vi "T Test.vi"(6 "alternative hypothesis":i32(ring) items=["mean(pop) != mean"=0, "mean(pop) > mean"=1, "mean(pop) < mean"=-1], 9 "significance level":dbl=0.05, 10 "mean":dbl, 11 "sample set":dbl[](array[numeric])) -> (0 "error":i32, 1 "confidence interval":cluster{"low":dbl, "high":dbl}={"low"=0.8260722090132093, "high"=0.8260722090132093} {"high" format="%.6g"; "low" format="%.6g"}, 2 "p value":dbl=0.05 format="%.6g", 3 "reject null hypothesis":bool, 4 "t test info":T1 {"sample t value" format="%_6g"; "t value" format="%_6g"; "sample se mean" format="%_6g"; "sample std" format="%_6g"; "sample mean" format="%_6g"})   [LabVIEW 2018, in "NI_Gmath.lvlib"]
doc: "Tests hypotheses about the <B>mean</B> of a population whose distribution is at least approximately normal but whose variance is unknown."
uses:
  NI_Gmath.lvlib
  st_t_control.ctl
  NI_AALBase.lvlib
panel:
  # "T Test\n(single sample set)"
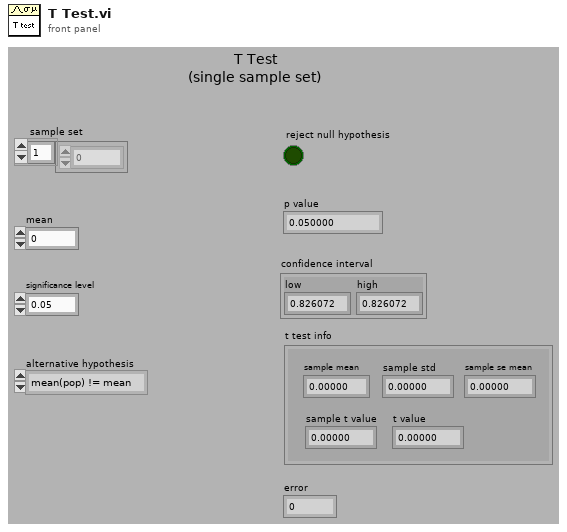
[diagram p1: front panel]
types:
  T1 = typedef "NI_Gmath.lvlib/st_t_control.ctl" = cluster{"sample mean":dbl, "sample std":dbl, "sample se mean":dbl, "sample t value":dbl, "t value":dbl}
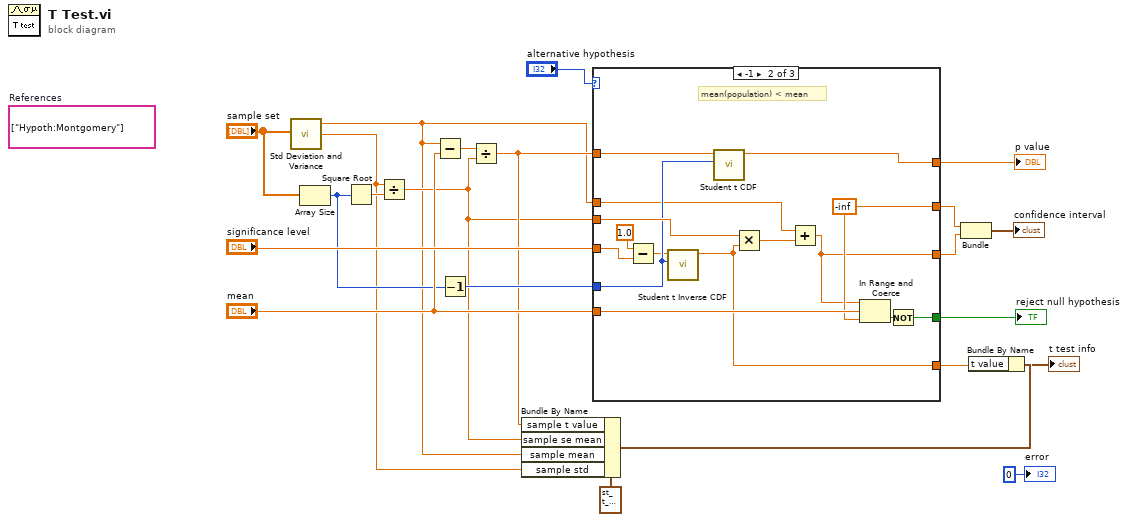
[diagram p0: block diagram]
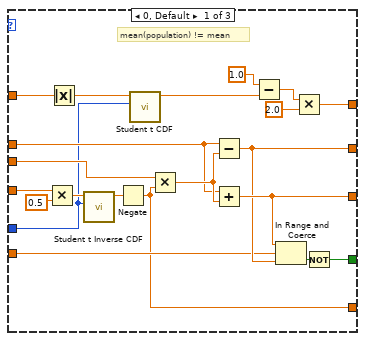
[diagram p2: hidden frame]
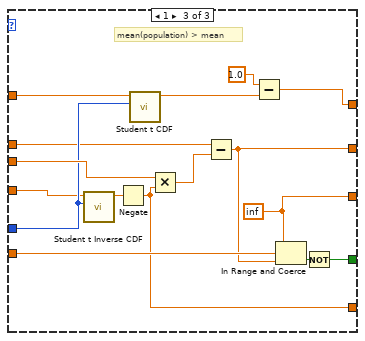
[diagram p3: hidden frame]
diagram:
  (unwired) string[] ["Hypoth:Montgomery"]  # References
  n1 = call "Std Deviation and Variance.vi"("X"="sample set") -> ("mean"=w1:dbl, "standard deviation"=w9:dbl)  [unwired: 1 in, 1 out]
  n2 = Array Size(array="sample set") -> (size(s)=w10:i32)
  n3 = Square Root(x=w10) -> (sqrt(x)=w11:dbl)
  n4 = Divide(x=w9, y=w11) -> (x/y=w7:dbl)
  n5 = Subtract(x=w1, y="mean") -> (x-y=w21:dbl)
  n6 = Decrement(x=w10) -> (x-1=w18:i32)
  n7 = Divide(x=w21, y=w7) -> (x/y=w8:dbl)
  n8 = Bundle By Name(cluster=T1 {"sample mean"=0.0, "sample std"=0.0, "sample se mean"=0.0, "sample t value"=0.0, "t value"=0.0} ("t test info"), "sample t value"=w8, "sample se mean"=w7, "sample mean"=w1, "sample std"=w9) -> (w6:T1)
  n9 = case shown="-1" "alternative hypothesis" {
    tunnel: "significance level" -> [w42 w50 w65]
    tunnel: w18 -> [w31 w54 w69]
    tunnel: w7 -> [w41 w58 w74]
    tunnel: [w37 w45 w62] -> w17
    tunnel: [w36 w46 w63] -> w16
    tunnel: [w34 w55 w71] -> w15
    tunnel: "mean" -> [w33 w53 w70]
    tunnel: w1 -> [w32 w52 w64]
    tunnel: w8 -> [w30 w47 w68]
    tunnel: [w25 w44 w61] -> w12
    tunnel: [w24 w48 w59] -> w4
    frame 0, Default {
      # "mean(population) != mean"
      n10 = Multiply(x=w42, y=0.5) -> (x*y=w38:dbl)
      n11 = Absolute Value(x=w30) -> (abs(x)=w23:dbl)
      n12 = call "Student t Inverse CDF.vi"("k degrees of freedom"=w31, "cdf(x)"=w38) -> ("x"=w39:dbl)  [unwired: 8 in, 1 out]
      n13 = Negate(x=w39) -> (-x=w24:dbl)
      n14 = call "Student t CDF.vi"("k degrees of freedom"=w31, "x"=w23) -> ("cdf(x)"=w28:dbl)  [unwired: 7 in, 2 out]
      n15 = Multiply(x=w41, y=w24) -> (x*y=w40:dbl)
      n16 = Subtract(x=w32, y=w40) -> (x-y=w36:dbl)
      n17 = Add(x=w32, y=w40) -> (x+y=w37:dbl)
      n18 = Subtract(x=1.0, y=w28) -> (x-y=w26:dbl)
      n19 = In Range and Coerce(upper limit=w37, x=w33, lower limit=w36) -> (In Range?=w35:bool)  [unwired: 1 out]
      n20 = Multiply(x=w26, y=2.0) -> (x*y=w25:dbl)
      n21 = Not(x=w35) -> (.not. x?=w34:bool)
    }
    frame -1 {
      w46 = -inf ("lower limit")
      # "mean(population) < mean"
      n22 = Subtract(x=1.0, y=w50) -> (x-y=w49:dbl)
      n23 = call "Student t Inverse CDF.vi"("k degrees of freedom"=w54, "cdf(x)"=w49) -> ("x"=w48:dbl)  [unwired: 8 in, 1 out]
      n24 = call "Student t CDF.vi"("k degrees of freedom"=w54, "x"=w47) -> ("cdf(x)"=w44:dbl)  [unwired: 7 in, 2 out]
      n25 = Multiply(x=w58, y=w48) -> (x*y=w57:dbl)
      n26 = Add(x=w52, y=w57) -> (x+y=w45:dbl)
      n27 = In Range and Coerce(upper limit=w45, x=w53, lower limit=w46) -> (In Range?=w56:bool)  [unwired: 1 out]
      n28 = Not(x=w56) -> (.not. x?=w55:bool)
    }
    frame 1 {
      w62 = inf
      # "mean(population) > mean"
      n29 = call "Student t Inverse CDF.vi"("k degrees of freedom"=w69, "cdf(x)"=w65) -> ("x"=w60:dbl)  [unwired: 8 in, 1 out]
      n30 = Negate(x=w60) -> (-x=w59:dbl)
      n31 = call "Student t CDF.vi"("k degrees of freedom"=w69, "x"=w68) -> ("cdf(x)"=w66:dbl)  [unwired: 7 in, 2 out]
      n32 = Multiply(x=w74, y=w59) -> (x*y=w73:dbl)
      n33 = Subtract(x=w64, y=w73) -> (x-y=w63:dbl)
      n34 = Subtract(x=1.0, y=w66) -> (x-y=w61:dbl)
      n35 = In Range and Coerce(upper limit=w62, x=w70, lower limit=w63) -> (In Range?=w72:bool)  [unwired: 1 out]
      n36 = Not(x=w72) -> (.not. x?=w71:bool)
    }
  }
  "reject null hypothesis" <- w15
  "p value" <- w12
  n37 = Bundle("lower limit"=w16, w17) -> (→"confidence interval":cluster{"lower limit":dbl, dbl})  [unwired: 1 in]
  n38 = Bundle By Name(cluster=w6, "t value"=w4) -> (→"t test info":T1)
  "error" <- 0 ("error")
